vi "counter 1.vi"() -> ()   [LabVIEW 2009]
panel:
  out "Compte 1":i32
  out "total cumulatif":i32
  in  "stop":bool
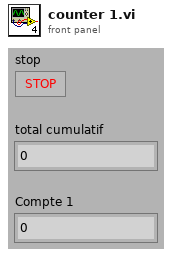
[diagram p1: front panel]
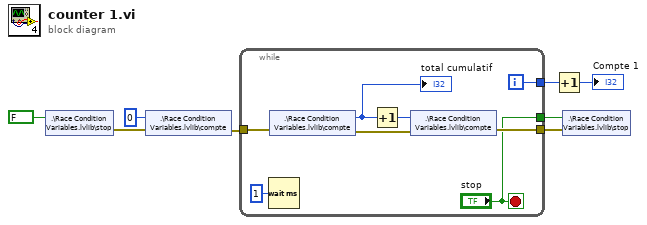
[diagram p0: block diagram]
diagram:
  n1 = shared-variable ".\\Race Condition Variables.lvlib\\stop"(FALSE ("stop")) -> (error out=w3:errorcluster)  [unwired: 1 in]
  n2 = shared-variable ".\\Race Condition Variables.lvlib\\compte"(0 ("counter"), error in=w3) -> (error out=w8:errorcluster)
  n3 = while "Boucle While" {
    tunnel: [w15] -> w7
    tunnel: w8 -> [w14]
    tunnel: [w10] -> w1
    tunnel: ["stop"] -> w2
    i -> [w15]
    stop <- "stop" stop-if-true
    n4 = Wait (ms) ("Attendre (ms)")(milliseconds to wait=u32 1) -> ()  [unwired: 1 out]
    n5 = shared-variable ".\\Race Condition Variables.lvlib\\compte"(error in=w14) -> (w11:i32, error out=w16:errorcluster)
    "total cumulatif" <- w11
    n6 = Increment ("Incrémenter")(x=w11) -> (x+1=w12:i32)
    n7 = shared-variable ".\\Race Condition Variables.lvlib\\compte"(w12, error in=w16) -> (error out=w10:errorcluster)
  }
  n8 = Increment ("Incrémenter")(x=w7) -> (x+1=→"Compte 1":i32)
  n9 = shared-variable ".\\Race Condition Variables.lvlib\\stop"(w2, error in=w1) -> ()  [unwired: 1 out]
